vi "QA.vi"(8 "ERRIN":errorcluster caption="entrée d'erreur (pas d'erreur)") -> (0 "ERROUT":errorcluster caption="sortie d'erreur", 2 "DATAOUT":string)   [LabVIEW 2020]
uses:
  OP300-CONTI-AUTO/VG/VG_ATEQ.vi
panel:
  in  "buffer d'écriture":string
  # "<\\B20\\BE:(A\\CC\\A9:P\\D2\\C5SS\\C9\\CFN\\A0HAU\\D4\\C5\\8D\\n"
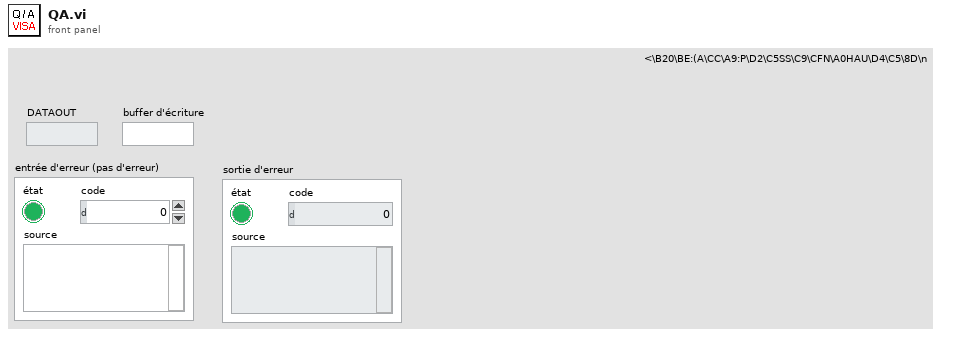
[diagram p1: front panel]
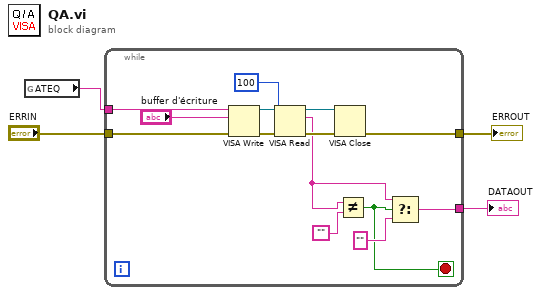
[diagram p0: block diagram]
diagram:
  n1 = global read "VG_ATEQ.vi" "ATEQ"() -> (w2:string)
  n2 = while {
    tunnel: [w18] -> w4
    tunnel: [w17] -> w3
    tunnel: "ERRIN" -> [w6]
    tunnel: w2 -> [w5]
    stop <- w7 stop-if-true
    n3 = VISA Write(VISA resource name=w5, write buffer="buffer d'écriture", error in (no error)=w6) -> (VISA resource name out=w12:refnum<visa-resource-name>, error out=w14:errorcluster)  [unwired: 1 out]
    n4 = VISA Read(VISA resource name=w12, byte count=u32 100 ("nombre d'octets"), error in (no error)=w14) -> (VISA resource name out=w15:refnum<visa-resource-name>, read buffer=w9:string, error out=w16:errorcluster)  [unwired: 1 out]
    n5 = VISA Close(VISA resource name=w15, error in (no error)=w16) -> (error out=w18:errorcluster)
    n6 = Not Equal?(x=w9, y="") -> (x != y?=w7:bool)
    n7 = Select(t=w9, s=w7, f="") -> (s? t:f=w17:string)
  }
  "ERROUT" <- w4
  "DATAOUT" <- w3
